vi "MT Apply Matched Filter (FSK).vi"(0 "input complex waveform":T1={"t0"=0.0, "dt"=1.0, "Y"=[]} {"Y" format="%.3f"; "dt" format="%^.2e"; "t0" format="%.4f"}, 5 "matched filter coefficients":dbl[](array[numeric]) format="%^.2e", 7 "samples per symbol (16)":i32=16, 11 "error in (no error)":errorcluster, 12 "symbol phase continuity":enum16{"continuous", "discontinuous"}(ring), 13 "reset? (T)":bool=TRUE) -> (4 "output phase waveform":cluster{"t0":dbl, "dt":dbl, "Y":dbl[]} {"Y" min=0.0 max=127.0 format="%.3f"; "dt" format="%^.2e"; "t0" format="%.4f"}, 15 "error out":errorcluster)   [LabVIEW 2020, in "niDMT.lvlib"]
doc: "This polymorphic instance applies a matched filter to an input FSK-modulated waveform. The VI first performs phase differentiation, followed by matched filtering on the phase of the <B>input complex waveform. </B>"
uses:
  <vilib>/addons/Modulation/niDMT.lvlib
  <vilib>/addons/Modulation/Analog/controls/Complex Data Waveform.ctl
  <vilib>/addons/Modulation/niAMT.lvlib
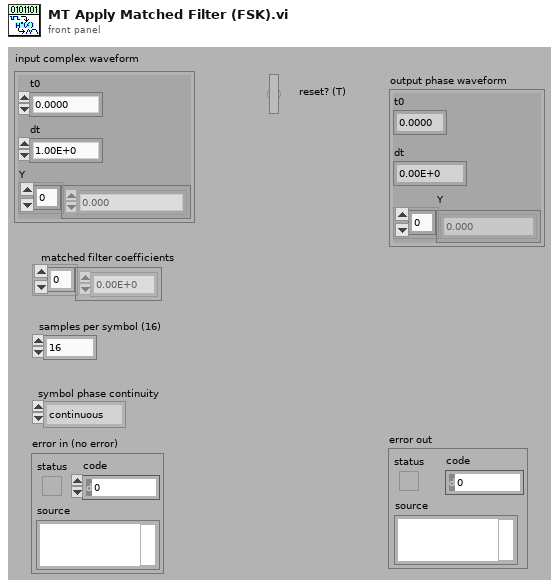
[diagram p1: front panel]
types:
  T1 = typedef "niAMT.lvlib/Complex Data Waveform.ctl" = cluster{"t0":dbl, "dt":dbl, "Y":cdb[]}
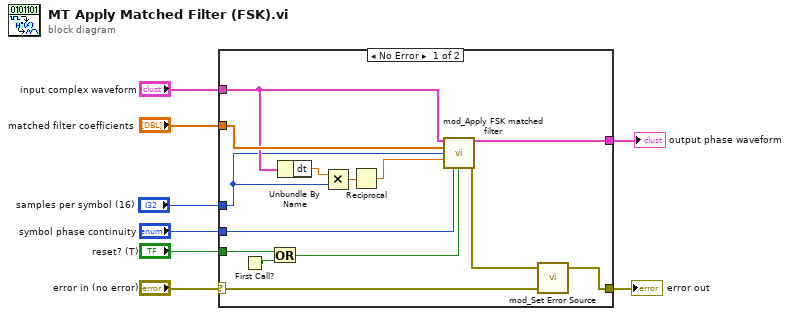
[diagram p0: block diagram]
diagram:
  n1 = case shown="No Error" "error in (no error)" {
    selector: "error in (no error)" -> [w9 w23]
    tunnel: "input complex waveform" -> [w16 _]
    tunnel: [w11 w23] -> w3
    tunnel: "matched filter coefficients" -> [w20 _]
    tunnel: "reset? (T)" -> [w22 _]
    tunnel: [w18 _] -> w4
    tunnel: "samples per symbol (16)" -> [w14 _]
    tunnel: "symbol phase continuity" -> [w17 _]
    frame No Error {
      n2 = First Call?() -> (First Call?: T/F=w21:bool)
      n3 = Or(x=w22, y=w21) -> (x .or. y?=w19:bool)
      n4 = Unbundle By Name(w16) -> ("dt"=w15:dbl)
      n5 = Multiply(x=w15, y=w14) -> (x*y=w13:dbl)
      n6 = Reciprocal(x=w13) -> (1/x=w12:dbl)
      n7 = call <vilib>:"mod_Apply FSK matched filter.vi"("input complex waveform"=w16, "matched filter coefficients"=w20, "samples per symbol (16)"=w14, "symbol rate, hz"=w12, "symbol phase continuity"=w17, "reset? (T)"=w19) -> ("output phase waveform"=w18:cluster{"t0":dbl, "dt":dbl, "Y":dbl[]}, "error out"=w10:errorcluster)  [unwired: 1 in, 7 out]
      n8 = call <vilib>:"mod_Set Error Source.vi"("initial error in (no error)"=w9, "final error in (no error)"=w10) -> ("error out"=w11:errorcluster)  [unwired: 3 out]
    }
    frame Error {
    }
  }
  "output phase waveform" <- w4
  "error out" <- w3
